vi "I2C CCC Example.vi"() -> ()   [LabVIEW 2018]
uses:
  <vilib>/Rock Robotics/SystemInterfaces/i2clib/i2c_bus.ctl
  library/Interface/Pixy Com.lvclass
  deviceSupport/FRC/I2C/RoboRIO I2C.lvclass
  library/Pixy2.lvlib
panel:
  in  "Device Address":u8=84 format="%.0x"
  in  "I2C Bus":T1
  out "error out":errorcluster
  in  "signature map":u8=255 format="%.0x"
  in  "max blocks":u8=255
  out "view":picture
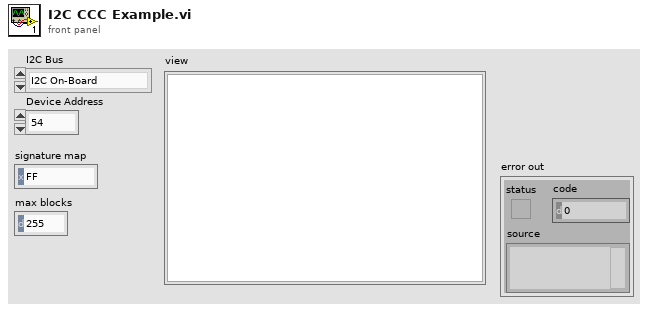
[diagram p1: front panel]
types:
  T1 = typedef "i2c_bus.ctl" = enum16{"I2C On-Board", "I2C MXP", "Invalid"}
  T2 = typedef "Pixy2.lvlib/Block.ctl" = cluster{"signature":u16, "x":u16, "y":u16, "width":u16, "height":u16, "angle":i16, "index":u8, "age":u8}
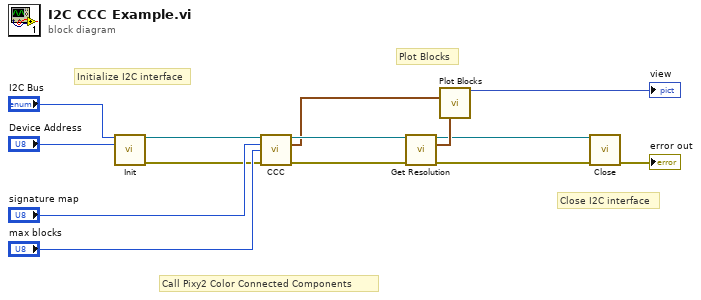
[diagram p0: block diagram]
diagram:
  # "Close I2C interface"
  # "Plot Blocks"
  # "Call Pixy2 Color Connected Components"
  # "Initialize I2C interface"
  n1 = call "Init.vi"("I2C Bus"="I2C Bus", "Device Address"="Device Address") -> ("comm interface out"=w5:refnum<class "Pixy Com.lvclass">, "error out"=w4:errorcluster)  [unwired: 12 in]
  n2 = call "CCC.vi"("comm interface in"=w5, "signature map"="signature map", "max blocks"="max blocks", "error in"=w4) -> ("comm interface out"=w10:refnum<class "Pixy Com.lvclass">, "blocks"=w8:T2[], "error out"=w11:errorcluster)  [unwired: 9 in]
  n3 = call "Get Resolution.vi"("comm interface in"=w10, "error in"=w11) -> ("comm interface out"=w2:refnum<class "Pixy Com.lvclass">, "resolution"=w12:cluster{"width":u16, "height":u16}, "error out"=w3:errorcluster)  [unwired: 11 in]
  n4 = call "Plot Blocks.vi"("blocks"=w8, "pixy resolution"=w12) -> ("picture out"=→"view":picture)  [unwired: 13 in]
  n5 = call-dynamic "Close.vi"("comm interface in"=w2, "error in"=w3) -> ("error out"=→"error out":errorcluster)  [unwired: 13 in]
